vi "Delete Path Node.vi"(6 "Child ID":i32[](array[numeric]), 8 "Parent ID":i32, 9 "ID":i16, 10 "Node To Index Lookup Map":map{i16, i16[]}(c390), 11 "Tree":T1[](array[typedef])) -> (2 "map out":map{i16, i16[]}(c390), 3 "Tree Out":T1[](array[typedef]))   [LabVIEW 2025]
uses:
  Types/Sequencing Tree Node.ctl
  Types/Single Cmd Info.ctl
  <vilib>/picture/picture.llb/imagedata.ctl
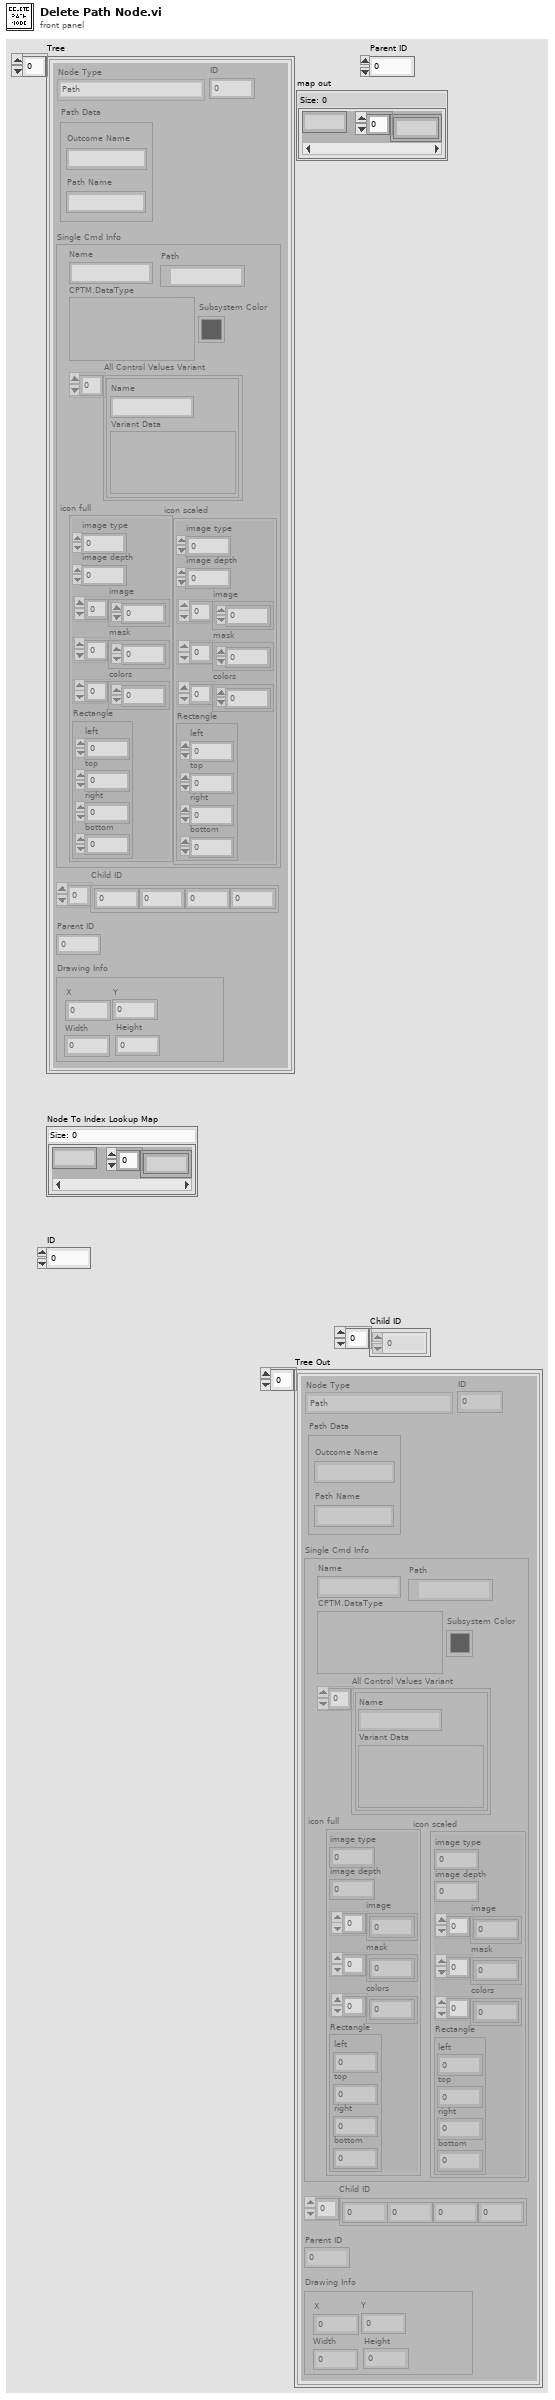
[diagram p1: front panel]
types:
  T1 = typedef "Sequencing Tree Node.ctl" = cluster{"Node Type":enum16{"Path", "Command", "Leaf"}, "ID":i16, "Path Data":cluster{"Path Name":string, "Outcome Name":string}, "Single Cmd Info":T2, "Child ID":i32[], "Parent ID":i32, "Drawing Info":cluster{"X":i32, "Y":i32, "Width":i32, "Height":i32}}
  T2 = typedef "Single Cmd Info.ctl" = cluster{"Name":string, "CPTM.DataType":variant, "All Control Values Variant":cluster{"Name":string, "Variant Data":variant}[], "icon full":T3, "icon scaled":T3, "Path":path, "Subsystem Color":u32}
  T3 = typedef "imagedata.ctl" = cluster{"image type":i32, "image depth":i32, "image":u8[], "mask":u8[], "colors":u32[], "Rectangle":cluster{"left":i16, "top":i16, "right":i16, "bottom":i16}}
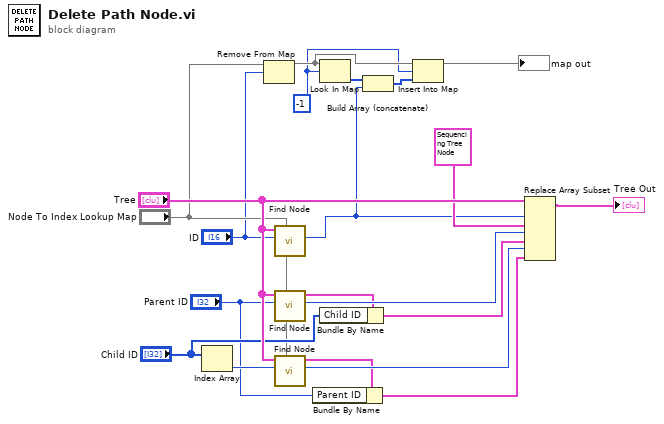
[diagram p0: block diagram]
diagram:
  w1 = i16 -1 ("key")
  n1 = Index Array(array="Child ID") -> (element=w17:i32)  [unwired: 1 in]
  n2 = Remove From Map(10:"ID", 11:"Node To Index Lookup Map") -> (3:w4:map{i16, i16[]})  [unwired: 2 out]
  n3 = call "Find Node.vi"("Node To Index Lookup Map"="Node To Index Lookup Map", "ID"="ID", "Tree"="Tree") -> ("Index"=w6:i16)  [unwired: 7 in, 1 out]
  n4 = call "Find Node.vi"("Node To Index Lookup Map"="Node To Index Lookup Map", "ID"="Parent ID", "Tree"="Tree") -> ("Index"=w19:i16, "Node"=w15:T1)  [unwired: 7 in]
  n5 = call "Find Node.vi"("Node To Index Lookup Map"="Node To Index Lookup Map", "ID"=w17, "Tree"="Tree") -> ("Index"=w20:i16, "Node"=w13:T1)  [unwired: 7 in]
  n6 = Bundle By Name(cluster=w13, "Parent ID"="Parent ID") -> (w11:T1)
  n7 = Look In Map(map=w4, key=w1) -> (value=w7:i16[])  [unwired: 1 in, 1 out]
  n8 = Bundle By Name(cluster=w15, "Child ID"="Child ID") -> (w10:T1)
  n9 = Build Array (concatenate)(w7, w6) -> (w5:i16[])
  n10 = Insert Into Map(map in=w4, key=w1, value=w5) -> (map out=→"map out":map{i16, i16[]})  [unwired: 2 out]
  n11 = Replace Array Subset(array="Tree", new element #1=T1 {"Node Type"=enum."Path", "ID"=-1, "Path Data"={"Path Name"="", "Outcome Name"=""}, "Single Cmd Info"={"Name"="", "CPTM.DataType"=variant, "All Control Values Variant"=[], "icon full"={"image type"=0, "image depth"=0, "image"=[], "mask"=[], "colors"=[], "Rectangle"={"left"=0, "top"=0, "right"=0, "bottom"=0}}, "icon scaled"={"image type"=0, "image depth"=0, "image"=[], "mask"=[], "colors"=[], "Rectangle"={"left"=0, "top"=0, "right"=0, "bottom"=0}}, "Path"=path "", "Subsystem Color"=16777216}, "Child ID"=[], "Parent ID"=0, "Drawing Info"={"X"=0, "Y"=0, "Width"=0, "Height"=0}} ("new element/subarray"), index #1=w6, new element #2=w10, index #2=w19, new element #3=w11, index #3=w20) -> (→"Tree Out":T1[])
